vi "Populate CD Child Nodes.vi"(8 "error in":errorcluster, 11 "StateValues":T1) -> (0 "error out":errorcluster)   [LabVIEW 2025]
uses:
  <resource>/objmgr/DOMUserDefRef.rc
  Shared/Types/NodeFilteringOptions.ctl
  Types/TD NodeRef Map Action.ctl
  Types/CD NodeRef Map Action.ctl
  Types/StateValues.ctl
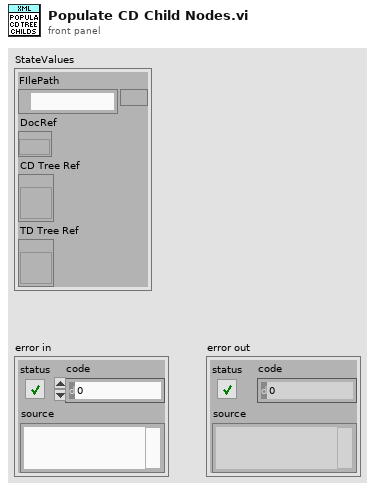
[diagram p1: front panel]
types:
  T1 = typedef "StateValues.ctl" = cluster{"FIlePath":path, "DocRef":refnum<k20>, "CD Tree Ref":refnum<vi>, "TD Tree Ref":refnum<vi>}
  T2 = typedef "NodeFilteringOptions.ctl" = enum16{"GetCustomDeviceNode", "GetAllChannelNodes", "GetAllSectionNodes", "GetAllWaveformNodes", "GetFirstChannelNode", "GetFirstSectionNode", "GetFirstWaveformNode", "GetSpecificSectionNode", "GetSpecificCustomDeviceNode", "GetSpecificChannelNode", "GetSpecificWaveformNode", "GetMatchedNamedNode", "GetEnumDefinitionsNode", "GetSpecificEnumDefinitionNode", "GetAllEnumDefinitionNodes", "GetDynamicChannelNodes"}
  T3 = typedef "CD NodeRef Map Action.ctl" = enum16{"Init", "Add XMLNodeRef", "Update ParentName", "Delete XMLNodeRef", "Get All Keys", "Get", "skip"}
  T4 = typedef "TD NodeRef Map Action.ctl" = enum16{"Init", "Add XMLNodeRef", "Delete XMLNodeRef", "Add TDNodeRefs", "Delete TDNodeRefs", "Clear TDNodeRefs", "Add ChildXMLNodeRef", "Delete ChildXMLNodeRef", "Get All Keys", "Update ParentName", "Get", "skip"}
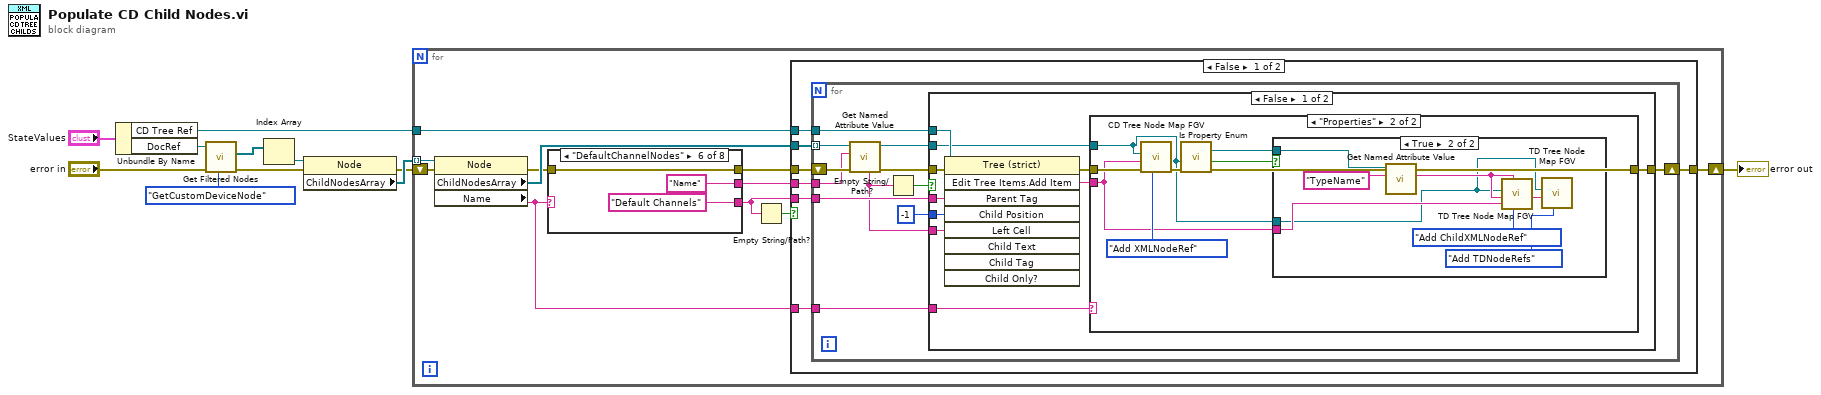
[diagram p0: block diagram]
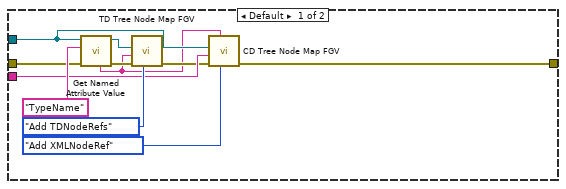
[diagram p2: hidden frame]
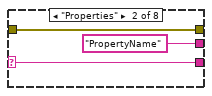
[diagram p7: hidden frame]
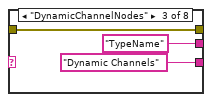
[diagram p8: hidden frame]
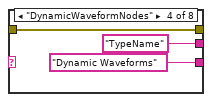
[diagram p9: hidden frame]
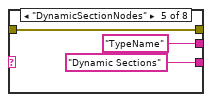
[diagram p10: hidden frame]
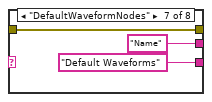
[diagram p11: hidden frame]
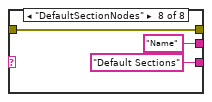
[diagram p12: hidden frame]
diagram:
  n1 = Unbundle By Name("StateValues") -> ("CD Tree Ref"=w2:refnum<vi>, "DocRef"=w3:refnum<k20>)
  n2 = call "Get Filtered Nodes.vi"("Node Filtering"=NodeFilteringOptions."GetCustomDeviceNode", "error in"="error in", "Document in"=w3) -> ("error out"=w6:errorcluster, "Filtered Nodes"=w10:refnum<k20>[])  [unwired: 4 in, 3 out]
  n3 = Index Array(array=w10) -> (element=w9:refnum<k20>)  [unwired: 1 in]
  n4 = property class="Node"(reference=w9, error in=w6) -> (error out=w7:errorcluster, "ChildNodesArray"=w8:refnum<k20>[])  [unwired: 1 out]
  n5 = for {
    tunnel: w8 -> [w22] mode=indexing
    shift-right: [w19] -> w5
    shift-left: w7 -> [w21]
    tunnel: w2 -> [w13]
    n6 = property class="Node"(reference=w22, error in=w21) -> (error out=w17:errorcluster, "ChildNodesArray"=w20:refnum<k20>[], "Name"=w12:string)  [unwired: 1 out]
    n7 = case shown="\"DefaultChannelNodes\"" w12 {
      selector: w12 -> [_ w82 _ _ _ _ _ _]
      tunnel: [_ w82 "Dynamic Channels" ("Attribute Name") "Dynamic Waveforms" ("Attribute Name") "Dynamic Sections" ("Attribute Name") "Default Channels" ("Attribute Name") "Default Waveforms" ("Attribute Name") "Default Sections" ("Attribute Name")] -> w15
      tunnel: [_ "PropertyName" ("Attribute Name") "TypeName" ("Attribute Name") "TypeName" ("Attribute Name") "TypeName" ("Attribute Name") "Name" ("Attribute Name") "Name" ("Attribute Name") "Name" ("Attribute Name")] -> w18
      tunnel: w17 -> [w79 w80 w85 w88 w91 w93 w96 w99]
      tunnel: [w79 w80 w85 w88 w91 w93 w96 w99] -> w16
      frame Default {
      }
      frame "Properties" {
      }
      frame "DynamicChannelNodes" {
      }
      frame "DynamicWaveformNodes" {
      }
      frame "DynamicSectionNodes" {
      }
      frame "DefaultChannelNodes" {
      }
      frame "DefaultWaveformNodes" {
      }
      frame "DefaultSectionNodes" {
      }
    }
    n8 = Empty String/Path?(string/path=w15) -> (empty?=w14:bool)
    n9 = case shown="False" w14 {
      tunnel: w20 -> [w29 _]
      tunnel: [w28 w78] -> w19
      tunnel: w18 -> [w27 _]
      tunnel: w16 -> [w26 w78]
      tunnel: w15 -> [w25 _]
      tunnel: w13 -> [w24 _]
      tunnel: w12 -> [w23 _]
      frame False {
        n10 = for {
          tunnel: w29 -> [w40] mode=indexing
          shift-right: [w38] -> w28
          shift-left: w26 -> [w41]
          tunnel: w25 -> [w36]
          tunnel: w27 -> [w35]
          tunnel: w24 -> [w32]
          tunnel: w23 -> [w30]
          n11 = call "Get Named Attribute Value.vi"("error in"=w41, "Attribute Name"=w35, "Node In"=w40) -> ("error out"=w39:errorcluster, "Node Out"=w31:refnum<k20>, "Attribute Value"=w34:string)  [unwired: 5 in, 1 out]
          n12 = Empty String/Path?(string/path=w34) -> (empty?=w33:bool)
          n13 = case shown="False" w33 {
            tunnel: w39 -> [w50 w77]
            tunnel: [w46 w77] -> w38
            tunnel: -1 ("Child Position") -> [w48 _]
            tunnel: w36 -> [w49 _]
            tunnel: w34 -> [w47 _]
            tunnel: w32 -> [w51 _]
            tunnel: w31 -> [w44 _]
            tunnel: w30 -> [w43 _]
            frame False {
              n14 = invoke class="Tree (strict)" method="Edit Tree Items.Add Item"(reference=w51, error in=w50, "Parent Tag"=w49, "Child Position"=w48, "Left Cell"=w47) -> (error out=w45:errorcluster, "Edit Tree Items:Add Item"=w42:string)  [unwired: 4 in, 7 out]
              n15 = case shown="\"Properties\"" w43 {
                tunnel: [w53 w65] -> w46
                tunnel: w45 -> [w55 w69]
                tunnel: w44 -> [w57 w63]
                tunnel: w42 -> [w56 w64]
                frame Default {
                  n16 = call "Get Named Attribute Value.vi"("error in"=w55, "Attribute Name"="TypeName", "Node In"=w57) -> ("error out"=w60:errorcluster, "Node Out"=w61:refnum<k20>, "Attribute Value"=w52:string)  [unwired: 5 in, 1 out]
                  n17 = call "TD Tree Node Map FGV.vi"("Action"=TD_NodeRef_Map_Action."Add TDNodeRefs", "error in"=w60, "Node Name"=w52, "Attribute Node"=w61) -> ("error out"=w54:errorcluster)  [unwired: 2 in, 5 out]
                  n18 = call "CD Tree Node Map FGV.vi"("Action"=CD_NodeRef_Map_Action."Add XMLNodeRef", "Parent Name in"=w52, "error in"=w54, "Node Name"=w56, "Attribute Node"=w57) -> ("error out"=w53:errorcluster)  [unwired: 2 in, 4 out]
                }
                frame "Properties" {
                  n19 = call "CD Tree Node Map FGV.vi"("Action"=CD_NodeRef_Map_Action."Add XMLNodeRef", "error in"=w69, "Node Name"=w64, "Attribute Node"=w63) -> ("error out"=w65:errorcluster)  [unwired: 3 in, 4 out]
                  n20 = call "Is Property Enum.vi"("error in"=w65, "Node"=w63) -> ("Is Enum Property"=w67:bool, "Enum Node"=w66:refnum<k20>)  [unwired: 7 in, 1 out]
                  n21 = case shown="True" w67 {
                    tunnel: w63 -> [_ w70]
                    tunnel: w64 -> [_ w75]
                    tunnel: w66 -> [_ w74]
                    frame False {
                    }
                    frame True {
                      n22 = call "Get Named Attribute Value.vi"("Attribute Name"="TypeName", "Node In"=w74) -> ("Attribute Value"=w72:string)  [unwired: 6 in, 3 out]
                      n23 = call "TD Tree Node Map FGV.vi"("Action"=TD_NodeRef_Map_Action."Add ChildXMLNodeRef", "Parent Node"=w72, "Node Name"=w75, "Attribute Node"=w70) -> ()  [unwired: 2 in, 6 out]
                      n24 = call "TD Tree Node Map FGV.vi"("Action"=TD_NodeRef_Map_Action."Add TDNodeRefs", "Node Name"=w72, "Attribute Node"=w70) -> ()  [unwired: 3 in, 6 out]
                    }
                  }
                }
              }
            }
            frame True {
            }
          }
        }
      }
      frame True {
      }
    }
  }
  "error out" <- w5
